vi "ReadSettings.vi"(8 "error in (no error)":errorcluster, 11 "Controller in":refnum<class "Controller.lvclass">) -> (0 "error out":errorcluster, 2 "Settings":T1, 3 "Controller out":refnum<class "Controller.lvclass">)   [LabVIEW 2024, in "GUI.lvlib" / "Controller.lvclass"]
uses:
  Controller.lvclass
  TypeDefs/Settings.ctl
  Controller.lvclass/Controller.ctl
  <vilib>/drjdpowell/SQLite Library/SQL Connection/Execute SQL (Single String).vi
  <vilib>/drjdpowell/SQLite Library/SQLite.lvlib
  <vilib>/drjdpowell/SQLite Library/SQL Connection/Connection.lvclass
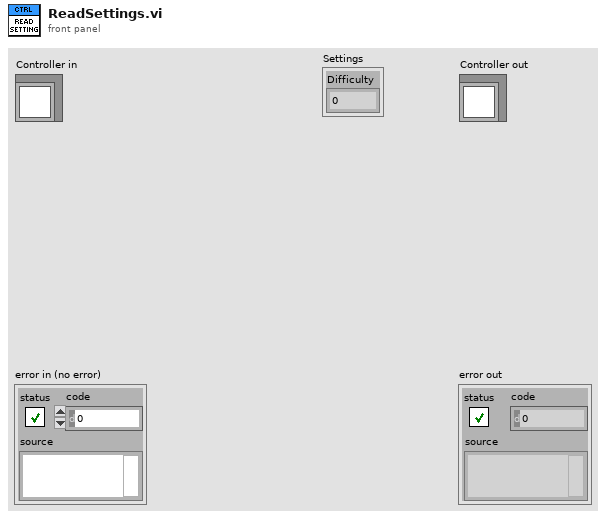
[diagram p1: front panel]
types:
  T1 = typedef "Settings.ctl" = cluster{"Difficulty":i32}
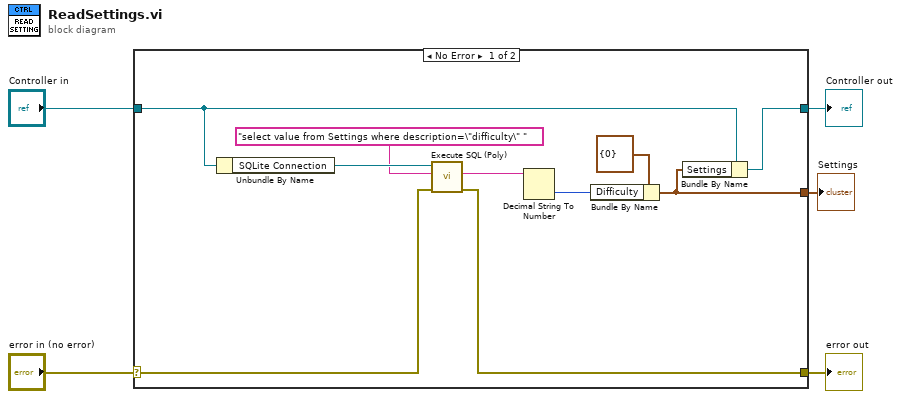
[diagram p0: block diagram]
diagram:
  n1 = case shown="No Error" "error in (no error)" {
    selector: "error in (no error)" -> [w13 w17]
    tunnel: [w12 w17] -> w4
    tunnel: [w6 w16] -> w2
    tunnel: "Controller in" -> [w8 w16]
    tunnel: [w7 _] -> w1
    frame No Error {
      n2 = Unbundle By Name(w8) -> ("SQLite Connection"=w15:refnum<class "Connection.lvclass">)
      n3 = call-poly <vilib>:"Execute SQL (Poly).vi"("error in (no error)"=w13, "SQL"="select value from Settings where description=\"difficulty\" ", "SQLite Connection in"=w15) -> ("error out"=w12:errorcluster, "Result"=w11:string)  [unwired: 6 in, 1 out]
      n4 = Decimal String To Number(string=w11) -> (number=w9:i32)  [unwired: 2 in, 1 out]
      n5 = Bundle By Name(cluster=T1 {"Difficulty"=0} ("Settings"), "Difficulty"=w9) -> (w7:T1)
      n6 = Bundle By Name(cluster=w8, "Settings"=w7) -> (w6:refnum<class "Controller.lvclass">)
    }
    frame Error {
    }
  }
  "error out" <- w4
  "Controller out" <- w2
  "Settings" <- w1
